vi "Read Digital Voltmeter History.vi"(8 "error in (no error)":errorcluster, 11 "VISA resource name":refnum<visa-resource-name>) -> (0 "error out":errorcluster, 1 "Minimum Value":dbl, 2 "Maximum Value":dbl, 3 "VISA resource name out":refnum<visa-resource-name>, 5 "Average Value":dbl)   [LabVIEW 2017, in "Scope.lvlib" / "Tektronix DPO MSO 2000 4000 Series.lvlib"]
doc: "Reads the readout value for the Digital Voltmeter function over the history period.\n\n<B>Notes:</B>\n(1) This VI is available for MDO3000 Series only.\n\n(2) Requires option MDO3DVM to be installed."
uses:
  Tektronix DPO MSO 2000 4000 Series.lvlib
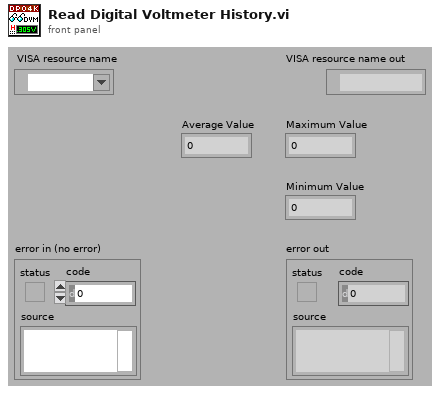
[diagram p1: front panel]
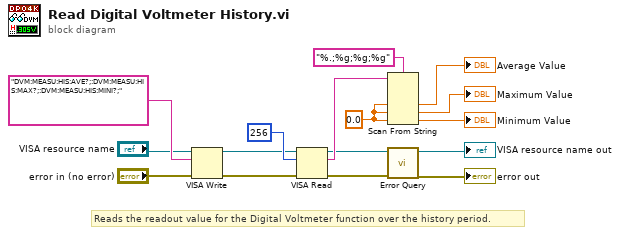
[diagram p0: block diagram]
diagram:
  w6 = 0.0 ("default value 1")
  # "Reads the readout value for the Digital Voltmeter function over the history period."
  n1 = VISA Write(VISA resource name="VISA resource name", write buffer="DVM:MEASU:HIS:AVE?;:DVM:MEASU:HIS:MAX?;:DVM:MEASU:HIS:MINI?;", error in (no error)="error in (no error)") -> (VISA resource name out=w2:refnum<visa-resource-name>, error out=w1:errorcluster)  [unwired: 1 out]
  n2 = VISA Read(VISA resource name=w2, byte count=u32 256, error in (no error)=w1) -> (VISA resource name out=w8:refnum<visa-resource-name>, read buffer=w12:string, error out=w7:errorcluster)  [unwired: 1 out]
  n3 = Scan From String(format string="%.;%g;%g;%g", input string=w12, default 1=w6, default 2=w6, default 3=w6) -> (output 1=→"Average Value":dbl, output 2=→"Maximum Value":dbl, output 3=→"Minimum Value":dbl)  [unwired: 2 in, 3 out]
  n4 = call "Error Query.vi"("error in (no error)"=w7, "VISA resource name"=w8) -> ("error out"=→"error out":errorcluster, "VISA resource name out"=→"VISA resource name out":refnum<visa-resource-name>)  [unwired: 6 in, 2 out]
